vi "[del]Firmware_Update.vi"(8 "error in (no error)":errorcluster) -> (0 "error out":errorcluster, 2 "Success":bool)   [LabVIEW 2011, in "CAN FD.lvlib"]
uses:
  CAN FD.lvlib
  bin/zlgcan.dll
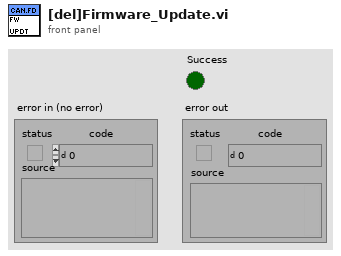
[diagram p1: front panel]
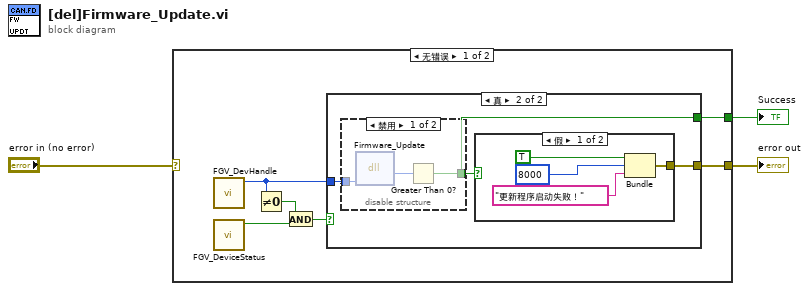
[diagram p0: block diagram]
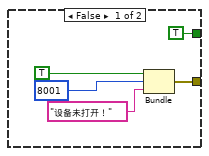
[diagram p2: hidden frame]
diagram:
  n1 = case shown="无错误" "error in (no error)" {
    selector: "error in (no error)" -> [_ w25]
    tunnel: [w5 w25] -> w3
    tunnel: [w4 _] -> w2
    frame No Error {
      n2 = call "FGV_DevHandle.vi"() -> ("handle out"=w6:u32)  [unwired: 9 in, 2 out]
      n3 = call "FGV_DeviceStatus.vi"() -> ("Open?"=w9:bool)  [unwired: 10 in, 1 out]
      n4 = Not Equal To 0?(x=w6) -> (x != 0?=w8:bool)
      n5 = And(x=w8, y=w9) -> (x .and. y?=w7:bool)
      n6 = case shown="真" w7 {
        tunnel: w6 -> [_ w17]
        tunnel: [w11 w16] -> w5
        tunnel: [TRUE w15] -> w4
        frame False {
          n7 = Bundle("status"=TRUE, "code"=8001, "消息"="设备未打开！") -> (w11:cluster{"status":bool, "code":i32, "消息":string})  [unwired: 1 in]
        }
        frame True {
          n8 = disable-structure shown="禁用" {
            disable-tunnel: w17 -> [w20 _]
            disable-tunnel: [w18 _] -> w15
            frame Disabled {
              n9 = dll-call lib="C:/Users/binck/Desktop/[CODE]USBCAN/CANFD Tool/bin/zlgcan.dll" fn="Firmware_Update"("device_handle"=w20) -> ("return"=w19:u32)  [unwired: 4 in, 2 out]
              n10 = Greater Than 0?(x=w19) -> (x > 0?=w18:bool)
            }
            frame Enabled {
            }
          }
          n11 = case shown="假" w15 {
            tunnel: [w21 _] -> w16
            frame False {
              n12 = Bundle("status"=TRUE, "code"=8000, "消息"="更新程序启动失败！") -> (w21:cluster{"status":bool, "code":i32, "消息":string})  [unwired: 1 in]
            }
            frame True {
            }
          }
        }
      }
    }
    frame Error {
    }
  }
  "Success" <- w2
  "error out" <- w3
